vi "Fdx Get Monitor Queue Status.vi"(8 "error in":errorcluster, 10 "QueueId":u32, 11 "InstrumentHandle_port":u32) -> (0 "error out":errorcluster, 1 "QueueStatus":T1 {"QueueStatus" items=["FDX_MON_STAT_EMPTY", "FDX_MON_STAT_ FILLED", "FDX_MON_STAT_ FULL", "FDX_MON_STAT_ OVERFLOW", "FDX_MON_STAT_ ERROR"]}, 2 "QueueIdOut":u32, 3 "InstrumentHandle_port":u32)   [LabVIEW 2020, in "AIM664LV.lvlib"]
uses:
  AIM664LV.lvlib
  AFDX_LibraryAdmin/FdxGlobalDllPath.vi
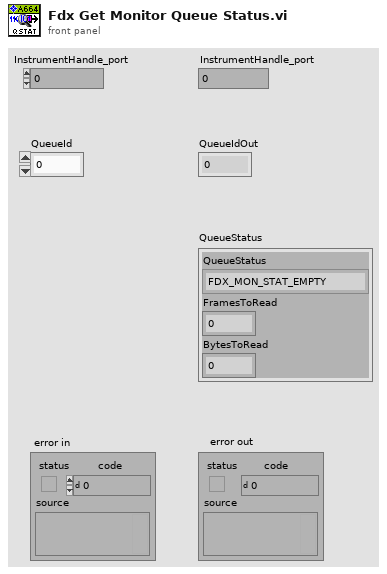
[diagram p1: front panel]
types:
  T1 = cluster{"QueueStatus":u32, "FramesToRead":u32, "BytesToRead":u32}
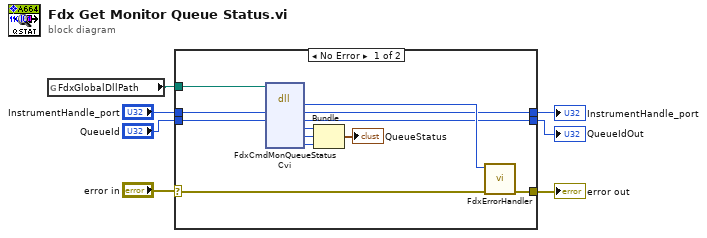
[diagram p0: block diagram]
diagram:
  n1 = global read "FdxGlobalDllPath.vi" "FdxGlobalDllPath"() -> (w5:path)
  n2 = case shown="No Error" "error in" {
    selector: "error in" -> [w18 w22]
    tunnel: [w19 w22] -> w7
    tunnel: w5 -> [w13 _]
    tunnel: "InstrumentHandle_port" -> [w11 w21]
    tunnel: [w10 w21] -> w3
    tunnel: "QueueId" -> [w9 w20]
    tunnel: [w8 w20] -> w1
    frame No Error {
      n3 = dll-call lib="aim_fdx.19.dll" fn="FdxCmdMonQueueStatusCvi"(path in=w13, "InstrumentHandle"=w11, "QueueId"=w9) -> ("status"=w17:i32, "InstrumentHandle"=w10:u32, "QueueId"=w8:u32, "QueueStatus"=w14:u32, "FramesToRead"=w15:u32, "BytesToRead"=w16:u32)  [unwired: 5 in, 2 out]
      n4 = Bundle("QueueStatus"=w14, "FramesToRead"=w15, "BytesToRead"=w16) -> (→"QueueStatus":T1)  [unwired: 1 in]
      n5 = call "FdxErrorHandler.vi"("error in"=w18, "AIM Error"=w17) -> ("error out"=w19:errorcluster)  [unwired: 9 in]
    }
    frame Error {
    }
  }
  "error out" <- w7
  "InstrumentHandle_port" <- w3
  "QueueIdOut" <- w1
